vi "Determine Periodic.vi"(4 "Period Reached?":bool, 5 "Start Time Offset Counts":u32, 6 "Generation Counter":u32, 7 "Start Time Offset":u32, 8 "Generation Iterations":u32, 9 "Generation Period":u32, 10 "Time Since Last Generation in":u32, 11 "Current Time":u32) -> (0 "Period Reached out":bool, 1 "Transmit":bool, 2 "Generation Counter out":u32, 3 "Time Since Last Generation out":u32)   [LabVIEW 2023, in "Protection and Counter Support Engine.lvlib"]
uses:
  Protection and Counter Support Engine.lvlib
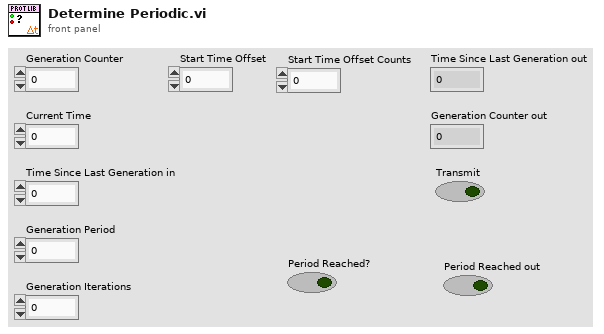
[diagram p1: front panel]
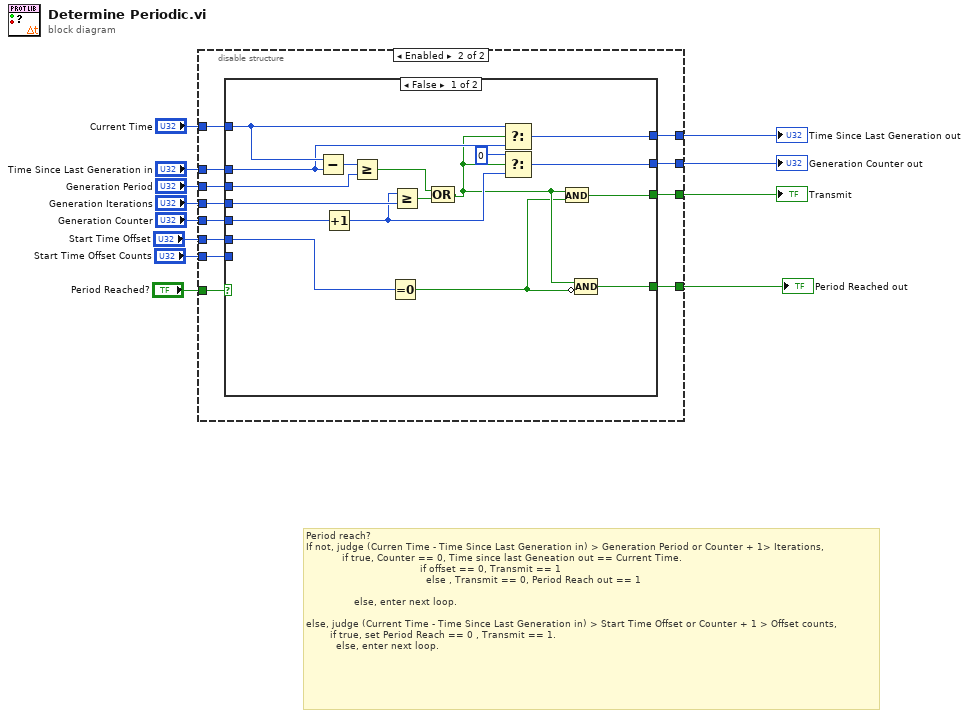
[diagram p0: block diagram]
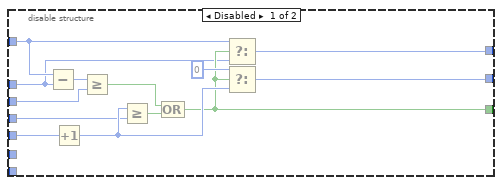
[diagram p2: hidden frame]
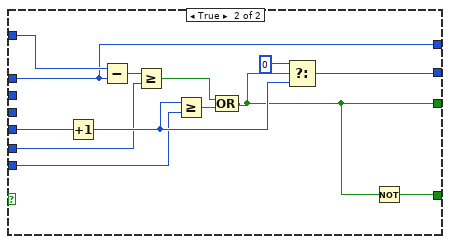
[diagram p3: hidden frame]
diagram:
  # "Period reach?\nIf not, judge (Curren Time - Time Since Last Generation in) > Generation Period or Counter + 1> Iterations, \n            if true, Counter == 0, Time since last Geneation out == Current Time.\n                                      if offset == 0, Transmit == 1\n                                        else , Transmit == 0, Period Reach out == 1     \n                         \n                else, enter next loop.\n\nelse, judge (Current Time - Time Since Last Generation in) > Start Time Offset or Counter + 1 > Offset counts,\n        if true, set Period Reach == 0 , Transmit == 1.\n          else, enter next loop."
  n1 = disable-structure shown="Enabled" {
    disable-tunnel: [w20 w37] -> w12
    disable-tunnel: [w19 w36] -> w11
    disable-tunnel: "Generation Iterations" -> [w18 w35]
    disable-tunnel: "Generation Counter" -> [w17 w34]
    disable-tunnel: [w16 w33] -> w8
    disable-tunnel: "Current Time" -> [w15 w32]
    disable-tunnel: "Time Since Last Generation in" -> [w14 w31]
    disable-tunnel: "Generation Period" -> [w13 w30]
    disable-tunnel: "Start Time Offset" -> [_ w28]
    disable-tunnel: "Start Time Offset Counts" -> [_ w27]
    disable-tunnel: "Period Reached?" -> [_ w29]
    disable-tunnel: [_ w26] -> w1
    frame Disabled {
      n2 = Subtract(x=w15, y=w14) -> (x-y=w21:u32)
      n3 = Increment(x=w17) -> (x+1=w24:u32)
      n4 = Greater Or Equal?(x=w21, y=w13) -> (x >= y?=w23:bool)
      n5 = Greater Or Equal?(x=w24, y=w18) -> (x >= y?=w22:bool)
      n6 = Compound Arithmetic op=OR(w23, w22) -> (w19:bool)
      n7 = Select(t=w15, s=w19, f=w14) -> (s? t:f=w16:u32)
      n8 = Select(t=u32 0, s=w19, f=w24) -> (s? t:f=w20:u32)
    }
    frame Enabled {
      n9 = case shown="False" w29 {
        tunnel: [w44 w60] -> w37
        tunnel: [w42 w55] -> w36
        tunnel: w35 -> [w51 _]
        tunnel: w34 -> [w50 w64]
        tunnel: [w43 w57] -> w33
        tunnel: w32 -> [w47 w62]
        tunnel: w31 -> [w46 w57]
        tunnel: w30 -> [w49 _]
        tunnel: w28 -> [w41 w59]
        tunnel: w27 -> [_ w58]
        tunnel: [w38 w56] -> w26
        frame False {
          n10 = Subtract(x=w47, y=w46) -> (x-y=w52:u32)
          n11 = Increment(x=w50) -> (x+1=w45:u32)
          n12 = Greater Or Equal?(x=w52, y=w49) -> (x >= y?=w54:bool)
          n13 = Equal To 0?(x=w41) -> (x = 0?=w39:bool)
          n14 = Greater Or Equal?(x=w45, y=w51) -> (x >= y?=w53:bool)
          n15 = Compound Arithmetic op=OR(w54, w53) -> (w40:bool)
          n16 = Select(t=w47, s=w40, f=w46) -> (s? t:f=w43:u32)
          n17 = Select(t=u32 0, s=w40, f=w45) -> (s? t:f=w44:u32)
          n18 = And(x=w40, y=w39) -> (x .and. y?=w42:bool)
          n19 = Compound Arithmetic op=AND(w40, invert w39) -> (w38:bool)
        }
        frame True {
          n20 = Increment(x=w64) -> (x+1=w61:u32)
          n21 = Subtract(x=w62, y=w57) -> (x-y=w65:u32)
          n22 = Greater Or Equal?(x=w65, y=w59) -> (x >= y?=w67:bool)
          n23 = Greater Or Equal?(x=w61, y=w58) -> (x >= y?=w66:bool)
          n24 = Compound Arithmetic op=OR(w67, w66) -> (w55:bool)
          n25 = Select(t=u32 0, s=w55, f=w61) -> (s? t:f=w60:u32)
          n26 = Not(x=w55) -> (.not. x?=w56:bool)
        }
      }
    }
  }
  "Generation Counter out" <- w12
  "Transmit" <- w11
  "Time Since Last Generation out" <- w8
  "Period Reached out" <- w1
